vi "Industrial Parameters FG.vi"(7 "Action":T2, 8 "error in (no error)":errorcluster, 10 "Parameters":T3, 11 "Node Ptr":T1 format="%.0x") -> (0 "error out":errorcluster, 2 "Parameters":T3, 3 "Item Ref out":T1=18446744073709551615 format="%.0x")   [LabVIEW 2019, in "Control Addon System Explorer.lvlib"]
uses:
  Control Addon System Explorer.lvlib
  <vilib>/NI VeriStand/Custom Device API/Custom Device Item Ref.ctl
  Addon Shared/Types/Industrial Parameters.ctl
  Types/Action.ctl
  Addon Shared/Constants.vi
  <vilib>/NI VeriStand/Custom Device API/Get Item Property (Boolean).vi
  <vilib>/NI VeriStand/Custom Device API/Get Item Property (Double).vi
  <vilib>/NI VeriStand/Custom Device API/Set Item Property (Boolean).vi
  <vilib>/NI VeriStand/Custom Device API/Set Item Property (Double).vi
  <vilib>/NI VeriStand/Custom Device API/Custom Device API.lvlib
  Addon Shared/Control Addon Shared.lvlib
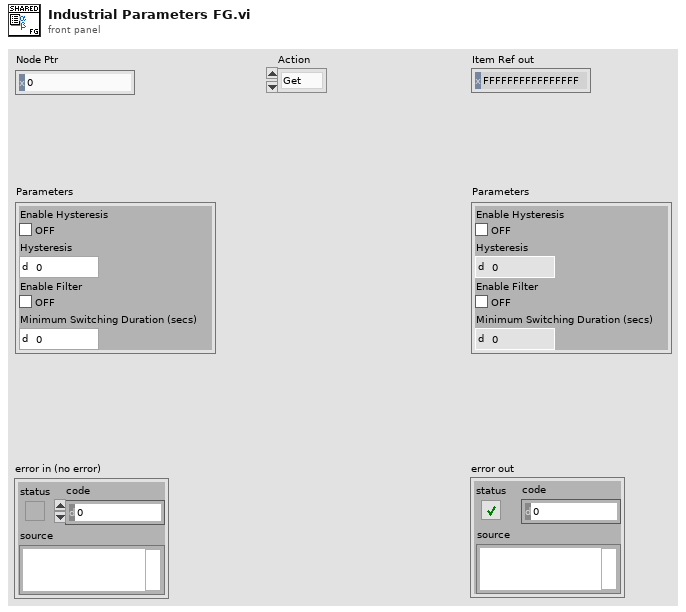
[diagram p1: front panel]
types:
  T1 = typedef "Custom Device API.lvlib/Custom Device Item Ref.ctl" = u64
  T2 = typedef "Control Addon System Explorer.lvlib/Action.ctl" = enum16{"Get", "Set"}
  T3 = typedef "Control Addon Shared.lvlib/Industrial Parameters.ctl" = cluster{"Enable Hysteresis":bool, "Hysteresis":dbl, "Enable Filter":bool, "Minimum Switching":dbl}
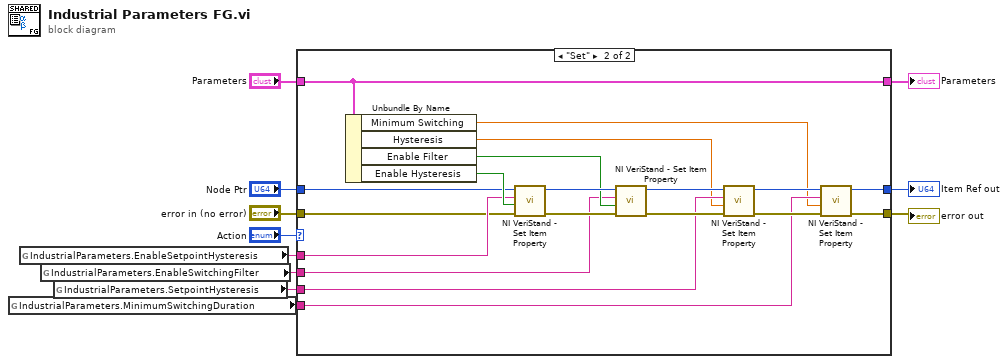
[diagram p0: block diagram]
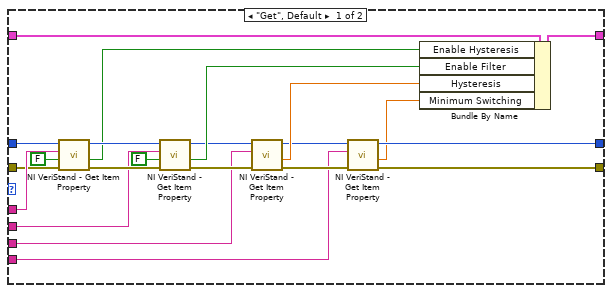
[diagram p2: hidden frame]
diagram:
  n1 = global read "Constants.vi" "IndustrialParameters.MinimumSwitchingDuration"() -> (w1:string)
  n2 = global read "Constants.vi" "IndustrialParameters.EnableSetpointHysteresis"() -> (w4:string)
  n3 = global read "Constants.vi" "IndustrialParameters.EnableSwitchingFilter"() -> (w3:string)
  n4 = global read "Constants.vi" "IndustrialParameters.SetpointHysteresis"() -> (w2:string)
  n5 = case shown="\"Set\"" "Action" {
    tunnel: "Node Ptr" -> [w26 w44]
    tunnel: "error in (no error)" -> [w27 w45]
    tunnel: "Parameters" -> [w33 w48]
    tunnel: [w32 w48] -> w7
    tunnel: [w15 w37] -> w5
    tunnel: [w14 w36] -> w6
    tunnel: w4 -> [w29 w47]
    tunnel: w3 -> [w28 w46]
    tunnel: w2 -> [w21 w41]
    tunnel: w1 -> [w13 w35]
    frame "Get", Default {
      n6 = call-poly <vilib>:"NI VeriStand - Get Item Property.vi"("error in (no error)"=w27, "Default Value"=FALSE, "Property Name"=w29, "Item Ref in"=w26) -> ("error out"=w31:errorcluster, "Value"=w25:bool, "Item Ref out"=w30:T1)  [unwired: 4 in, 1 out]
      n7 = call-poly <vilib>:"NI VeriStand - Get Item Property.vi"("error in (no error)"=w31, "Default Value"=FALSE, "Property Name"=w28, "Item Ref in"=w30) -> ("error out"=w22:errorcluster, "Value"=w24:bool, "Item Ref out"=w23:T1)  [unwired: 4 in, 1 out]
      n8 = call-poly <vilib>:"NI VeriStand - Get Item Property.vi"("error in (no error)"=w22, "Property Name"=w21, "Item Ref in"=w23) -> ("error out"=w16:errorcluster, "Value"=w18:dbl, "Item Ref out"=w17:T1)  [unwired: 5 in, 1 out]
      n9 = call-poly <vilib>:"NI VeriStand - Get Item Property.vi"("error in (no error)"=w16, "Property Name"=w13, "Item Ref in"=w17) -> ("error out"=w15:errorcluster, "Value"=w12:dbl, "Item Ref out"=w14:T1)  [unwired: 5 in, 1 out]
      n10 = Bundle By Name(cluster=w33, "Enable Hysteresis"=w25, "Enable Filter"=w24, "Hysteresis"=w18, "Minimum Switching"=w12) -> (w32:T3)
    }
    frame "Set" {
      n11 = Unbundle By Name(w48) -> ("Minimum Switching"=w34:dbl, "Hysteresis"=w40:dbl, "Enable Filter"=w49:bool, "Enable Hysteresis"=w50:bool)
      n12 = call-poly <vilib>:"NI VeriStand - Set Item Property.vi"("error in (no error)"=w45, "Value"=w50, "Property Name"=w47, "Item Ref in"=w44) -> ("error out"=w51:errorcluster, "Item Ref out"=w52:T1)  [unwired: 5 in, 1 out]
      n13 = call-poly <vilib>:"NI VeriStand - Set Item Property.vi"("error in (no error)"=w51, "Value"=w49, "Property Name"=w46, "Item Ref in"=w52) -> ("error out"=w43:errorcluster, "Item Ref out"=w42:T1)  [unwired: 5 in, 1 out]
      n14 = call-poly <vilib>:"NI VeriStand - Set Item Property.vi"("error in (no error)"=w43, "Value"=w40, "Property Name"=w41, "Item Ref in"=w42) -> ("error out"=w38:errorcluster, "Item Ref out"=w39:T1)  [unwired: 5 in, 1 out]
      n15 = call-poly <vilib>:"NI VeriStand - Set Item Property.vi"("error in (no error)"=w38, "Value"=w34, "Property Name"=w35, "Item Ref in"=w39) -> ("error out"=w37:errorcluster, "Item Ref out"=w36:T1)  [unwired: 5 in, 1 out]
    }
  }
  "Parameters" <- w7
  "Item Ref out" <- w6
  "error out" <- w5
